vi "TestCommunication.vi"() -> ()   [LabVIEW 2014]
panel:
  out "Error":bool
  in  "exit":bool
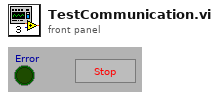
[diagram p1: front panel]
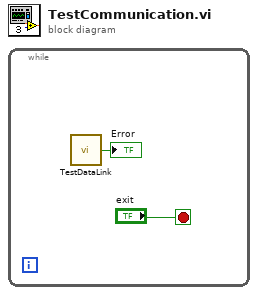
[diagram p0: block diagram]
diagram:
  n1 = while {
    stop <- "exit" stop-if-true
    n2 = call "TestDataLink.vi"() -> ("Error"=→"Error":bool)  [unwired: 2 in]
  }
